vi "Begin.vi"() -> (0 "CameraDevRef 2":T1, 1 "CameraDevRef":T1)   [LabVIEW 2011]
doc: "Called before other user functions, this VI is expected to open initial I/O refnums, load in file data, and do all program initialization. Notice that the <B>error out</B> terminal is simply used for data flow. Wiring it to other structures or subVIs ensures that this VI runs first."
uses:
  <vilib>/Rock Robotics/WPI/Camera/WPI_CameraDevRef.ctl
  <vilib>/Rock Robotics/SystemInterfaces/DIO/FPGA_DIOPWMChannel.ctl
  <vilib>/Rock Robotics/WPI/Joystick/WPI_JoystickDeviceEnum.ctl
  <vilib>/Rock Robotics/SystemInterfaces/AI/FPGA_AIChannel.ctl
  <vilib>/Rock Robotics/SystemInterfaces/DIO/FPGA_DIORelayChannel.ctl
  <vilib>/Rock Robotics/SystemInterfaces/DIO/FPGA_DIOChannel.ctl
  <vilib>/Rock Robotics/SystemInterfaces/AI/FPGA_AIGyroChannel.ctl
  <vilib>/Rock Robotics/WPI/Relay/WPI_RelayDirection.ctl
  <vilib>/Rock Robotics/WPI/Encoder/WPI_EncoderType.ctl
  <vilib>/Rock Robotics/WPI/DriverStation/DriverStationLCD/WPI_DriverStationLCDLCDLine.ctl
  <vilib>/Rock Robotics/WPI/MotorControl/WPI_MotorControlOpen Victor.vi
  <vilib>/Rock Robotics/WPI/MotorControl/WPI_MotorControlOpen Jaguar.vi
  Robot Global Data.vi
  <vilib>/Utility/file.llb/Read From Spreadsheet File (DBL).vi
  <vilib>/Rock Robotics/WPI/Counter/WPI_CounterDigitalInputToDigitalSource.vi
  <vilib>/Rock Robotics/SystemInterfaces/Typedef/FPGA_TypedefDigitalModule.ctl
  <vilib>/Rock Robotics/SystemInterfaces/Typedef/FPGA_TypedefAnalogModule.ctl
panel:
  out "Path and file":string
  in  "Balls In Robot At Start":dbl=2.0
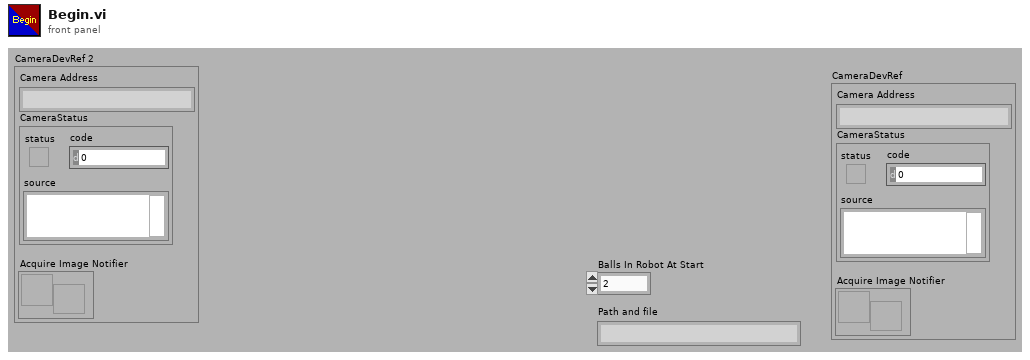
[diagram p1: front panel]
types:
  T1 = typedef "WPI_CameraDevRef.ctl" = cluster{"Camera Address":string, "CameraStatus":errorcluster, "Acquire Image Notifier":refnum<notifier>}
  T2 = typedef "FPGA_DIOPWMChannel.ctl" = enum8{"PWM 1", "PWM 2", "PWM 3", "PWM 4", "PWM 5", "PWM 6", "PWM 7", "PWM 8", "PWM 9", "PWM 10", "Invalid"}
  T3 = typedef "WPI_DriverStationLCDLCDLine.ctl" = enum16{"Main - Line 1", "User - Line 2", "User - Line 3", "User - Line 4", "User - Line 5", "User - Line 6"}
  T4 = typedef "WPI_EncoderType.ctl" = enum16{"1x", "2x", "4x"}
  T5 = typedef "FPGA_DIOChannel.ctl" = enum8{"DIO 1", "DIO 2", "DIO 3", "DIO 4", "DIO 5", "DIO 6", "DIO 7", "DIO 8", "DIO 9", "DIO 10", "DIO 11", "DIO 12", "DIO 13", "DIO 14", "Invalid"}
  T6 = typedef "FPGA_DIORelayChannel.ctl" = enum8{"Relay 1", "Relay 2", "Relay 3", "Relay 4", "Relay 5", "Relay 6", "Relay 7", "Relay 8", "Invalid"}
  T7 = typedef "WPI_RelayDirection.ctl" = enum16{"Both directions", "Forward only", "Reverse only"}
  T8 = typedef "FPGA_AIGyroChannel.ctl" = enum8{"AI 1", "AI 2", "Invalid"}
  T9 = typedef "FPGA_AIChannel.ctl" = enum8{"AI 1", "AI 2", "AI 3", "AI 4", "AI 5", "AI 6", "AI 7", "AI 8", "Invalid"}
  T10 = typedef "WPI_JoystickDeviceEnum.ctl" = enum16{"USB 1", "USB 2", "USB 3", "USB 4", "Kinect 1", "Kinect 2"}
  T11 = typedef "WPI_CameraImageSize.ctl" = enum16{"640x480", "320x240", "160x120"}
  T12 = cluster{"fps":i32, "compression":i32, "Image Size":T11}
  T13 = typedef "WPI_MotorControlDeviceRef.ctl" = cluster{"DeviceStatus":errorcluster, "Type":enum16{"PWM", "CAN"}, "PWM":cluster{"Digital Module":T14, "PWM Channel":T2, "DeadBand":T15}, "CAN":cluster{"Device Number":u8, "Control Mode":T16, "Semaphore":T17, "Max Vout":dbl}, "Invert":bool, "TransformRef":T18, "InvTransformRef":T18}
  T14 = typedef "FPGA_TypedefDigitalModule.ctl" = enum16{"Digital Module 1", "Digital Module 2"}
  T15 = typedef "WPI_PWMDeadband.ctl" = cluster{"Name":string, "maxPositivePwm":i32, "minPositivePwm":i32, "centerPwm":i32, "maxNegativePwm":i32, "minNegativePwm":i32, "angularRange":u16}
  T16 = typedef "WPI_CANJaguar_ControlMode.ctl" = enum8{"Percent VBus", "Current", "Speed", "Position", "Voltage"}
  T17 = typedef "Semaphore RefNum" = refnum<k1>
  T18 = typedef "WPI_PWMTransform_ConPane.ctl" = refnum<vi>
  T19 = typedef "WPI_ServoDeviceRef.ctl" = cluster{"DeviceStatus":errorcluster, "Digital Module":T14, "PWM Channel":T2, "DeadBand":T15}
  T20 = typedef "WPI_AnalogChannelDevRef.ctl" = cluster{"DevStatus":errorcluster, "Analog Module":T21, "Analog Channel":T9}
  T21 = typedef "FPGA_TypedefAnalogModule.ctl" = enum16{"Analog Module 1", "Analog Module 2"}
  T22 = typedef "WPI_CameraWhite Balance Values.ctl" = enum16{"Auto", "Fixed indoor", "Fixed outdoor 1", "Fixed outdoor 2", "Fixed fluorescent 1", "Fixed fluorescent 2", "Hold current"}
  T23 = typedef "WPI_JoystickDevRef.ctl" = cluster{"Device":T10}
  T24 = typedef "WPI_RelayDevRef.ctl" = cluster{"DevStatus":errorcluster, "Relay Channel":T6, "Digital Module":T14, "Relay Direction":T7}
  T25 = typedef "WPI_CameraExposure Values.ctl" = enum16{"Auto", "Flicker-free 50 Hz", "Flicker-free 60 Hz", "Hold current"}
  T26 = typedef "WPI_DigitalInputDevRef.ctl" = cluster{"DevStatus":errorcluster, "DIO Channel":T5, "Digital Module":T14}
  T27 = typedef "FPGA_CounterEncoderSourceConvertionLVSourceType.ctl" = cluster{"DevStatus":errorcluster, "AnalogTriggerMode?":bool, "DigitalMode":cluster{"Digital Module":T14, "DIO Channel":T28}, "AnalogTriggerMode":cluster{"AnalogTriggerIndex":T29, "OutputType":T30}}
  T28 = typedef "FPGA_DIODigitalSourceChannel.ctl" = enum8{"DIO 1", "DIO 2", "DIO 3", "DIO 4", "DIO 5", "DIO 6", "DIO 7", "DIO 8", "DIO 9", "DIO 10", "DIO 11", "DIO 12", "DIO 13", "DIO 14", "Disabled"}
  T29 = typedef "FPGA_AnalogTriggerIndex.ctl" = enum8{"Trig 0", "Trig 1", "Trig 2", "Trig 3", "Trig 4", "Trig 5", "Trig 6", "Trig 7", "Invalid"}
  T30 = typedef "FPGA_AnalogTriggerOutType.ctl" = enum16{"InWindow", "TriggerState", "Rising", "Falling"}
  T31 = typedef "WPI_EncoderDevRef.ctl" = cluster{"DevStatus":errorcluster, "EncoderIndex":T32, "CounterIndex":T33, "DistancePerCount":dbl, "Decoding Type":T4}
  T32 = typedef "FPGA_EncoderIdx.ctl" = enum8{"Enc 0", "Enc 1", "Enc 2", "Enc 3", "Invalid"}
  T33 = typedef "FPGA_CounterCtrSystemIndex.ctl" = enum8{"Ctr 0", "Ctr 1", "Ctr 2", "Ctr 3", "Ctr 4", "Ctr 5", "Ctr 6", "Ctr 7", "Invalid"}
  T34 = typedef "WPI_GyroDevRef.ctl" = cluster{"DevStatus":errorcluster, "Analog Module":T21, "Analog Channel":T9, "Offset":dbl, "Gain (VoltsPerDegree/Second)":dbl}
  T35 = typedef "WPI_UltrasonicDeviceRef.ctl" = cluster{"DevStatus":errorcluster, "Ping Digital Module":T14, "Echo Digital Module":T14, "Ping Channel":T5, "Echo Channel":T5, "CntIndex":T33}
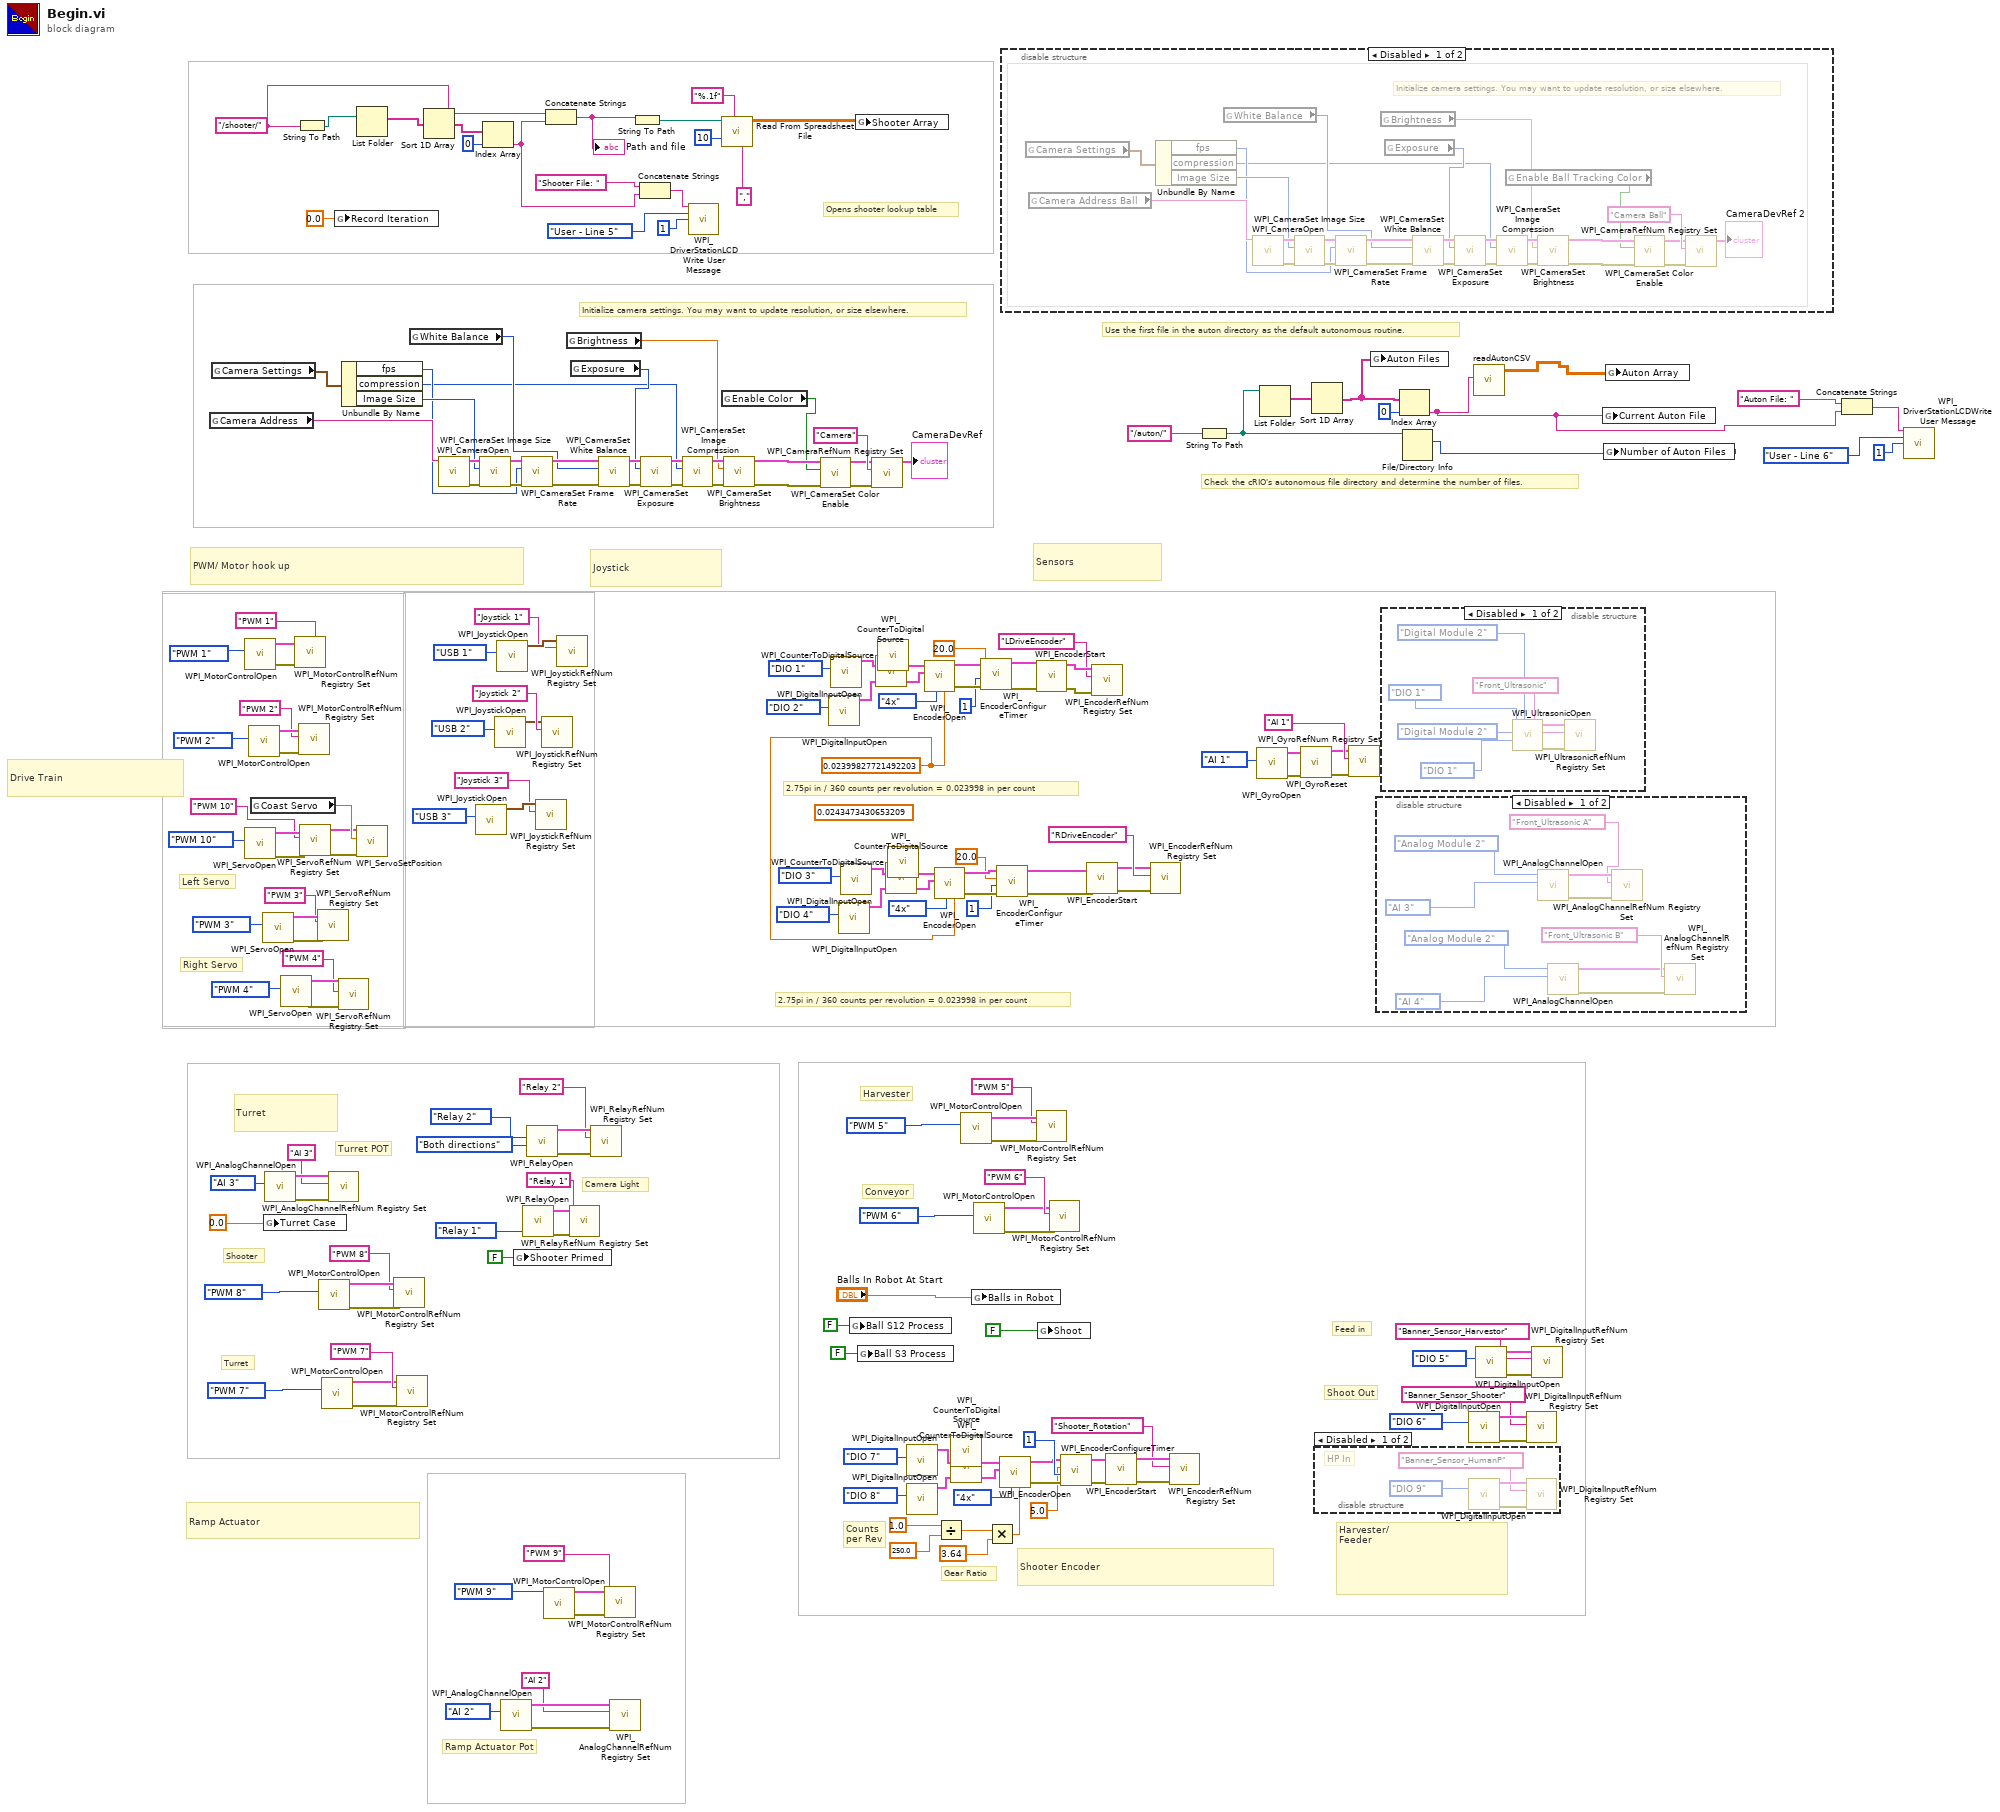
[diagram p0: block diagram]
diagram:
  (unwired) 0.0243473430653209 ("DistancePerCount")
  w39 = 0.02399827721492203 ("DistancePerCount")
  w87 = "/shooter/" ("string")
  # "Shooter Encoder"
  # "Counts\nper Rev"
  # "Gear Ratio"
  # "Check the cRIO's autonomous file directory and determine the number of files."
  # "Use the first file in the auton directory as the default autonomous routine."
  # "2.75pi in / 360 counts per revolution = 0.023998 in per count"
  # "2.75pi in / 360 counts per revolution = 0.023998 in per count"
  # "Opens shooter lookup table"
  # "Shoot Out"
  # "Feed in"
  # "Harvester"
  # "Conveyor"
  # "Shooter"
  # "Initialize camera settings. You may want to update resolution, or size elsewhere."
  # "Camera Light"
  # "Ramp Actuator Pot"
  # "Turret POT"
  # "Turret"
  # "Right Servo"
  # "Left Servo"
  # "Harvester/\nFeeder"
  # "Turret"
  # "Ramp Actuator"
  # "Drive Train"
  # "Sensors"
  # "Joystick"
  # "PWM/ Motor hook up"
  n1 = global read "Robot Global Data.vi" "Camera Address"() -> (w140:string)
  n2 = global read "Robot Global Data.vi" "Camera Settings"() -> (w139:T12)
  n3 = call-poly <vilib>:"WPI_MotorControlOpen.vi"("PWM Channel"=FPGA_DIOPWMChannel."PWM 1") -> ("error out"=w180:errorcluster, "MotorControlDeviceRef"=w182:T13)  [unwired: 9 in]
  n4 = call <vilib>:"WPI_ServoOpen.vi"("PWM Channel"=FPGA_DIOPWMChannel."PWM 10") -> ("error out"=w2:errorcluster, "ServoDeviceRef"=w6:T19)  [unwired: 9 in]
  n5 = call-poly <vilib>:"WPI_MotorControlOpen.vi"("PWM Channel"=FPGA_DIOPWMChannel."PWM 2") -> ("error out"=w178:errorcluster, "MotorControlDeviceRef"=w176:T13)  [unwired: 9 in]
  n6 = global read "Robot Global Data.vi" "Coast Servo"() -> (w7:dbl)
  n7 = call <vilib>:"WPI_ServoOpen.vi"("PWM Channel"=FPGA_DIOPWMChannel."PWM 3") -> ("error out"=w193:errorcluster, "ServoDeviceRef"=w198:T19)  [unwired: 9 in]
  n8 = global write "Robot Global Data.vi" "Turret Case"(0.0 ("Return To Home Case")) -> ()
  n9 = call <vilib>:"WPI_AnalogChannelOpen.vi"("Analog Channel"=FPGA_AIChannel."AI 3") -> ("error out"=w169:errorcluster, "AIDeviceRef"=w170:T20)  [unwired: 9 in]
  n10 = call <vilib>:"WPI_ServoOpen.vi"("PWM Channel"=FPGA_DIOPWMChannel."PWM 4") -> ("error out"=w192:errorcluster, "ServoDeviceRef"=w196:T19)  [unwired: 9 in]
  n11 = call <vilib>:"WPI_MotorControlRefNum Registry Set.vi"("error in (no error)"=w180, "refnum name"="PWM 1", "MotorControlDevRef"=w182) -> ()  [unwired: 7 in, 2 out]
  n12 = String To Path(string=w87) -> (path=w96:path)
  n13 = call <vilib>:"WPI_MotorControlRefNum Registry Set.vi"("error in (no error)"=w178, "refnum name"="PWM 2", "MotorControlDevRef"=w176) -> ()  [unwired: 7 in, 2 out]
  n14 = call <vilib>:"WPI_ServoRefNum Registry Set.vi"("error in (no error)"=w2, "refnum name"="PWM 10", "ServoDeviceRef"=w6) -> ("error out"=w3:errorcluster, "ServoDeviceRef"=w4:T19)  [unwired: 7 in]
  n15 = call <vilib>:"WPI_ServoRefNum Registry Set.vi"("error in (no error)"=w193, "refnum name"="PWM 3", "ServoDeviceRef"=w198) -> ()  [unwired: 7 in, 2 out]
  n16 = call-poly <vilib>:"WPI_MotorControlOpen.vi"("PWM Channel"=FPGA_DIOPWMChannel."PWM 8") -> ("error out"=w123:errorcluster, "MotorControlDeviceRef"=w125:T13)  [unwired: 9 in]
  n17 = call-poly <vilib>:"WPI_MotorControlOpen.vi"("PWM Channel"=FPGA_DIOPWMChannel."PWM 7") -> ("error out"=w174:errorcluster, "MotorControlDeviceRef"=w172:T13)  [unwired: 9 in]
  n18 = call <vilib>:"WPI_AnalogChannelRefNum Registry Set.vi"("error in (no error)"=w169, "refnum name"="AI 3", "AIDeviceRef"=w170) -> ()  [unwired: 7 in, 2 out]
  n19 = global write "Robot Global Data.vi" "Record Iteration"(0.0 ("Record Iteration")) -> ()
  n20 = call <vilib>:"WPI_ServoRefNum Registry Set.vi"("error in (no error)"=w192, "refnum name"="PWM 4", "ServoDeviceRef"=w196) -> ()  [unwired: 7 in, 2 out]
  n21 = Unbundle By Name(w139) -> ("fps"=w137:i32, "compression"=w134:i32, "Image Size"=w138:T11)
  n22 = List Folder(path=w96) -> (filenames=w95:string[])  [unwired: 1 in, 5 out]
  n23 = call <vilib>:"WPI_ServoSetPosition.vi"("error in (no error)"=w3, "Position"=w7, "ServoDeviceRef"=w4) -> ()  [unwired: 7 in, 2 out]
  n24 = call <vilib>:"WPI_MotorControlRefNum Registry Set.vi"("error in (no error)"=w123, "refnum name"="PWM 8", "MotorControlDevRef"=w125) -> ()  [unwired: 7 in, 2 out]
  n25 = call <vilib>:"WPI_MotorControlRefNum Registry Set.vi"("error in (no error)"=w174, "refnum name"="PWM 7", "MotorControlDevRef"=w172) -> ()  [unwired: 7 in, 2 out]
  n26 = global read "Robot Global Data.vi" "White Balance"() -> (w136:T22)
  n27 = Sort 1D Array(array=w95) -> (sorted array=w94:string[])
  n28 = call <vilib>:"WPI_CameraOpen.vi"("Camera Address"=w140) -> ("error out"=w146:errorcluster, "CameraDevRef"=w147:T1)  [unwired: 1 in, 8 out]
  n29 = call <vilib>:"WPI_JoystickOpen.vi"("JoystickDevice"=WPI_JoystickDeviceEnum."USB 3") -> ("JoystickDevRef"=w185:T23)  [unwired: 10 in]
  n30 = call <vilib>:"WPI_CameraSet Image Size.vi"("error in (no error)"=w146, "Image Size"=w138, "CameraDevRef"=w147) -> ("error out"=w145:errorcluster, "CameraDevRef Out"=w148:T1)  [unwired: 7 out]
  n31 = Index Array(array=w94, index=0) -> (element=w13:string)
  n32 = call <vilib>:"WPI_JoystickOpen.vi"("JoystickDevice"=WPI_JoystickDeviceEnum."USB 2") -> ("JoystickDevRef"=w188:T23)  [unwired: 10 in]
  n33 = call <vilib>:"WPI_JoystickOpen.vi"("JoystickDevice"=WPI_JoystickDeviceEnum."USB 1") -> ("JoystickDevRef"=w191:T23)  [unwired: 10 in]
  n34 = call <vilib>:"WPI_AnalogChannelOpen.vi"("Analog Channel"=FPGA_AIChannel."AI 2") -> ("error out"=w164:errorcluster, "AIDeviceRef"=w165:T20)  [unwired: 9 in]
  n35 = global write "Robot Global Data.vi" "Shooter Primed"(FALSE ("Ball S3 Process")) -> ()
  n36 = call <vilib>:"WPI_CameraSet Frame Rate.vi"("error in (no error)"=w145, "Frame Rate (fps)"=w137, "CameraDevRef"=w148) -> ("error out"=w144:errorcluster, "CameraDevRef Out"=w150:T1)  [unwired: 7 out]
  n37 = call <vilib>:"WPI_RelayOpen.vi"("Relay Channel"=FPGA_DIORelayChannel."Relay 1") -> ("error out"=w157:errorcluster, "RelayDevRef"=w156:T24)  [unwired: 9 in]
  n38 = call <vilib>:"WPI_RelayOpen.vi"("Relay Direction"=WPI_RelayDirection."Both directions", "Relay Channel"=FPGA_DIORelayChannel."Relay 2") -> ("error out"=w82:errorcluster, "RelayDevRef"=w83:T24)  [unwired: 8 in]
  n39 = call <vilib>:"WPI_JoystickRefNum Registry Set.vi"("refnum name"="Joystick 3", "JoystickDevRef"=w185) -> ()  [unwired: 8 in, 2 out]
  n40 = call <vilib>:"WPI_JoystickRefNum Registry Set.vi"("refnum name"="Joystick 2", "JoystickDevRef"=w188) -> ()  [unwired: 8 in, 2 out]
  n41 = call-poly <vilib>:"WPI_MotorControlOpen.vi"("PWM Channel"=FPGA_DIOPWMChannel."PWM 9") -> ("error out"=w160:errorcluster, "MotorControlDeviceRef"=w161:T13)  [unwired: 9 in]
  n42 = Concatenate Strings(w87, w13) -> (w89:string)
  "Path and file" <- w89
  n43 = call <vilib>:"WPI_JoystickRefNum Registry Set.vi"("refnum name"="Joystick 1", "JoystickDevRef"=w191) -> ()  [unwired: 8 in, 2 out]
  n44 = global read "Robot Global Data.vi" "Brightness"() -> (w133:dbl)
  n45 = call <vilib>:"WPI_RelayRefNum Registry Set.vi"("error in (no error)"=w157, "refnum name"="Relay 1", "RelayDevRef"=w156) -> ()  [unwired: 7 in, 2 out]
  n46 = global read "Robot Global Data.vi" "Exposure"() -> (w135:T25)
  n47 = call <vilib>:"WPI_RelayRefNum Registry Set.vi"("error in (no error)"=w82, "refnum name"="Relay 2", "RelayDevRef"=w83) -> ()  [unwired: 7 in, 2 out]
  n48 = call <vilib>:"WPI_CameraSet White Balance.vi"("error in (no error)"=w144, "White Balance"=w136, "CameraDevRef"=w150) -> ("error out"=w143:errorcluster, "CameraDevRef Out"=w149:T1)  [unwired: 7 out]
  n49 = call <vilib>:"WPI_MotorControlRefNum Registry Set.vi"("error in (no error)"=w160, "refnum name"="PWM 9", "MotorControlDevRef"=w161) -> ()  [unwired: 7 in, 2 out]
  n50 = call <vilib>:"WPI_AnalogChannelRefNum Registry Set.vi"("error in (no error)"=w164, "refnum name"="AI 2", "AIDeviceRef"=w165) -> ()  [unwired: 7 in, 2 out]
  n51 = String To Path(string=w89) -> (path=w88:path)
  n52 = Concatenate Strings("Shooter File: ", w13) -> (w11:string)
  n53 = call <vilib>:"WPI_CameraSet Exposure.vi"("error in (no error)"=w143, "Exposure"=w135, "CameraDevRef"=w149) -> ("error out"=w142:errorcluster, "CameraDevRef Out"=w152:T1)  [unwired: 7 out]
  n54 = call <vilib>:"WPI_CameraSet Image Compression.vi"("error in (no error)"=w142, "Compression"=w134, "CameraDevRef"=w152) -> ("error out"=w141:errorcluster, "CameraDevRef Out"=w151:T1)  [unwired: 7 out]
  n55 = call <vilib>:"WPI_DriverStationLCDWrite User Message.vi"("line text"=w11, "line"=WPI_DriverStationLCDLCDLine."User - Line 5", "starting column"=i8 1) -> ()  [unwired: 2 in, 11 out]
  n56 = call-poly <vilib>:"Read From Spreadsheet File.vi"("delimiter (\\t)"="," ("delimiter (\\t)"), "format (%.3f)"="%.1f", "number of rows (all:-1)"=10, "file path (dialog if empty)"=w88) -> ("all rows"=w86:dbl[][])  [unwired: 1 in, 6 out]
  n57 = global read "Robot Global Data.vi" "Enable Color"() -> (w128:bool)
  n58 = call <vilib>:"WPI_CameraSet Brightness.vi"("error in (no error)"=w141, "Brightness"=w133, "CameraDevRef"=w151) -> ("error out"=w131:errorcluster, "CameraDevRef Out"=w132:T1)  [unwired: 7 out]
  n59 = call <vilib>:"WPI_CameraSet Color Enable.vi"("error in (no error)"=w131, "Color Enabled"=w128, "CameraDevRef"=w132) -> ("error out"=w129:errorcluster, "CameraDevRef Out"=w130:T1)  [unwired: 7 in]
  n60 = call <vilib>:"WPI_DigitalInputOpen.vi"("DIO Channel"=FPGA_DIOChannel."DIO 2") -> ("DigitalInputDevRef"=w74:T26)  [unwired: 9 in, 1 out]
  n61 = call <vilib>:"WPI_DigitalInputOpen.vi"("DIO Channel"=FPGA_DIOChannel."DIO 1") -> ("DigitalInputDevRef"=w71:T26)  [unwired: 9 in, 1 out]
  n62 = call <vilib>:"WPI_DigitalInputOpen.vi"("DIO Channel"=FPGA_DIOChannel."DIO 4") -> ("DigitalInputDevRef"=w65:T26)  [unwired: 9 in, 1 out]
  n63 = call <vilib>:"WPI_DigitalInputOpen.vi"("DIO Channel"=FPGA_DIOChannel."DIO 3") -> ("DigitalInputDevRef"=w68:T26)  [unwired: 9 in, 1 out]
  n64 = global write "Robot Global Data.vi" "Ball S12 Process"(FALSE ("Ball S12 Process")) -> ()
  n65 = global write "Robot Global Data.vi" "Shooter Array"(w86) -> ()
  n66 = global write "Robot Global Data.vi" "Ball S3 Process"(FALSE ("Ball S3 Process")) -> ()
  n67 = call <vilib>:"WPI_CameraRefNum Registry Set.vi"("error in (no error)"=w129, "refnum name"="Camera", "CameraDevRef"=w130) -> ("CameraDevRef"=→"CameraDevRef":T1)  [unwired: 8 out]
  n68 = call-poly <vilib>:"WPI_CounterToDigitalSource.vi"("DigitalInputDevRef"=w74) -> ("Digital Source"=w75:T27)  [unwired: 6 in]
  n69 = call-poly <vilib>:"WPI_CounterToDigitalSource.vi"("DigitalInputDevRef"=w71) -> ("Digital Source"=w70:T27)  [unwired: 6 in]
  n70 = call-poly <vilib>:"WPI_CounterToDigitalSource.vi"("DigitalInputDevRef"=w65) -> ("Digital Source"=w64:T27)  [unwired: 6 in]
  n71 = call-poly <vilib>:"WPI_CounterToDigitalSource.vi"("DigitalInputDevRef"=w68) -> ("Digital Source"=w69:T27)  [unwired: 6 in]
  n72 = call <vilib>:"WPI_DigitalInputOpen.vi"("DIO Channel"=FPGA_DIOChannel."DIO 7") -> ("DigitalInputDevRef"=w23:T26)  [unwired: 9 in, 1 out]
  n73 = call <vilib>:"WPI_DigitalInputOpen.vi"("DIO Channel"=FPGA_DIOChannel."DIO 8") -> ("DigitalInputDevRef"=w26:T26)  [unwired: 9 in, 1 out]
  n74 = call <vilib>:"WPI_EncoderOpen.vi"("DistancePerCount"=w39, "Decoding Type"=WPI_EncoderType."4x", "BSource"=w75, "ASource"=w70) -> ("error out"=w43:errorcluster, "EncoderDevRef"=w46:T31)  [unwired: 6 in]
  n75 = call <vilib>:"WPI_EncoderOpen.vi"("DistancePerCount"=w39, "Decoding Type"=WPI_EncoderType."4x", "BSource"=w64, "ASource"=w69) -> ("error out"=w61:errorcluster, "EncoderDevRef"=w60:T31)  [unwired: 6 in]
  n76 = Divide(x=1.0, y=250.0) -> (x/y=w20:dbl)
  n77 = call-poly <vilib>:"WPI_CounterToDigitalSource.vi"("DigitalInputDevRef"=w23) -> ("Digital Source"=w22:T27)  [unwired: 6 in]
  n78 = call-poly <vilib>:"WPI_CounterToDigitalSource.vi"("DigitalInputDevRef"=w26) -> ("Digital Source"=w27:T27)  [unwired: 6 in]
  n79 = call-poly <vilib>:"WPI_MotorControlOpen.vi"("PWM Channel"=FPGA_DIOPWMChannel."PWM 5") -> ("error out"=w119:errorcluster, "MotorControlDeviceRef"=w121:T13)  [unwired: 9 in]
  n80 = global write "Robot Global Data.vi" "Balls in Robot"("Balls In Robot At Start") -> ()
  n81 = call-poly <vilib>:"WPI_MotorControlOpen.vi"("PWM Channel"=FPGA_DIOPWMChannel."PWM 6") -> ("error out"=w118:errorcluster, "MotorControlDeviceRef"=w116:T13)  [unwired: 9 in]
  n82 = call <vilib>:"WPI_EncoderConfigureTimer.vi"("error in (no error)"=w43, "Number Samples to Average"=u8 1, "Minimum Rate"=20.0, "EncoderDevRef"=w46) -> ("error out"=w44:errorcluster, "EncoderDevRef"=w45:T31)  [unwired: 6 in]
  n83 = Multiply(x=w20, y=3.64) -> (x*y=w18:dbl)
  n84 = call <vilib>:"WPI_EncoderConfigureTimer.vi"("error in (no error)"=w61, "Number Samples to Average"=u8 1, "Minimum Rate"=20.0, "EncoderDevRef"=w60) -> ("error out"=w57:errorcluster, "EncoderDevRef"=w58:T31)  [unwired: 6 in]
  n85 = call <vilib>:"WPI_EncoderOpen.vi"("DistancePerCount"=w18, "Decoding Type"=WPI_EncoderType."4x", "BSource"=w27, "ASource"=w22) -> ("error out"=w30:errorcluster, "EncoderDevRef"=w31:T31)  [unwired: 6 in]
  n86 = disable-structure shown="Disabled" {
    frame Disabled {
      # "Initialize camera settings. You may want to update resolution, or size elsewhere."
      n87 = global read "Robot Global Data.vi" "Camera Settings"() -> (w212:T12)
      n88 = global read "Robot Global Data.vi" "Camera Address Ball"() -> (w213:string)
      n89 = Unbundle By Name(w212) -> ("fps"=w210:i32, "compression"=w207:i32, "Image Size"=w211:T11)
      n90 = global read "Robot Global Data.vi" "White Balance"() -> (w209:T22)
      n91 = call <vilib>:"WPI_CameraOpen.vi"("Camera Address"=w213) -> ("error out"=w219:errorcluster, "CameraDevRef"=w220:T1)  [unwired: 1 in, 8 out]
      n92 = call <vilib>:"WPI_CameraSet Image Size.vi"("error in (no error)"=w219, "Image Size"=w211, "CameraDevRef"=w220) -> ("error out"=w218:errorcluster, "CameraDevRef Out"=w221:T1)  [unwired: 7 out]
      n93 = call <vilib>:"WPI_CameraSet Frame Rate.vi"("error in (no error)"=w218, "Frame Rate (fps)"=w210, "CameraDevRef"=w221) -> ("error out"=w217:errorcluster, "CameraDevRef Out"=w223:T1)  [unwired: 7 out]
      n94 = global read "Robot Global Data.vi" "Brightness"() -> (w206:dbl)
      n95 = global read "Robot Global Data.vi" "Exposure"() -> (w208:T25)
      n96 = call <vilib>:"WPI_CameraSet White Balance.vi"("error in (no error)"=w217, "White Balance"=w209, "CameraDevRef"=w223) -> ("error out"=w216:errorcluster, "CameraDevRef Out"=w222:T1)  [unwired: 7 out]
      n97 = call <vilib>:"WPI_CameraSet Exposure.vi"("error in (no error)"=w216, "Exposure"=w208, "CameraDevRef"=w222) -> ("error out"=w215:errorcluster, "CameraDevRef Out"=w225:T1)  [unwired: 7 out]
      n98 = call <vilib>:"WPI_CameraSet Image Compression.vi"("error in (no error)"=w215, "Compression"=w207, "CameraDevRef"=w225) -> ("error out"=w214:errorcluster, "CameraDevRef Out"=w224:T1)  [unwired: 7 out]
      n99 = global read "Robot Global Data.vi" "Enable Ball Tracking Color"() -> (w201:bool)
      n100 = call <vilib>:"WPI_CameraSet Brightness.vi"("error in (no error)"=w214, "Brightness"=w206, "CameraDevRef"=w224) -> ("error out"=w204:errorcluster, "CameraDevRef Out"=w205:T1)  [unwired: 7 out]
      n101 = call <vilib>:"WPI_CameraSet Color Enable.vi"("error in (no error)"=w204, "Color Enabled"=w201, "CameraDevRef"=w205) -> ("error out"=w202:errorcluster, "CameraDevRef Out"=w203:T1)  [unwired: 7 in]
      n102 = call <vilib>:"WPI_CameraRefNum Registry Set.vi"("error in (no error)"=w202, "refnum name"="Camera Ball", "CameraDevRef"=w203) -> ("CameraDevRef"=→"CameraDevRef 2":T1)  [unwired: 8 out]
    }
    frame Enabled {
    }
  }
  n103 = call <vilib>:"WPI_EncoderStart.vi"("error in (no error)"=w44, "EncoderDevRef"=w45) -> ("error out"=w78:errorcluster, "EncoderDevRef"=w77:T31)  [unwired: 8 in]
  n104 = call <vilib>:"WPI_MotorControlRefNum Registry Set.vi"("error in (no error)"=w119, "refnum name"="PWM 5", "MotorControlDevRef"=w121) -> ()  [unwired: 7 in, 2 out]
  n105 = global write "Robot Global Data.vi" "Shoot"(FALSE ("Ball S12 Process")) -> ()
  n106 = call <vilib>:"WPI_MotorControlRefNum Registry Set.vi"("error in (no error)"=w118, "refnum name"="PWM 6", "MotorControlDevRef"=w116) -> ()  [unwired: 7 in, 2 out]
  n107 = call <vilib>:"WPI_EncoderConfigureTimer.vi"("error in (no error)"=w30, "Number Samples to Average"=u8 1, "Minimum Rate"=5.0, "EncoderDevRef"=w31) -> ("error out"=w34:errorcluster, "EncoderDevRef"=w33:T31)  [unwired: 6 in]
  n108 = call <vilib>:"WPI_EncoderStart.vi"("error in (no error)"=w57, "EncoderDevRef"=w58) -> ("error out"=w55:errorcluster, "EncoderDevRef"=w56:T31)  [unwired: 8 in]
  n109 = call <vilib>:"WPI_EncoderRefNum Registry Set.vi"("error in (no error)"=w78, "refnum name"="LDriveEncoder", "EncoderDevRef"=w77) -> ()  [unwired: 7 in, 2 out]
  n110 = call <vilib>:"WPI_EncoderStart.vi"("error in (no error)"=w34, "EncoderDevRef"=w33) -> ("error out"=w36:errorcluster, "EncoderDevRef"=w35:T31)  [unwired: 8 in]
  n111 = call <vilib>:"WPI_EncoderRefNum Registry Set.vi"("error in (no error)"=w55, "refnum name"="RDriveEncoder", "EncoderDevRef"=w56) -> ()  [unwired: 7 in, 2 out]
  n112 = call <vilib>:"WPI_EncoderRefNum Registry Set.vi"("error in (no error)"=w36, "refnum name"="Shooter_Rotation", "EncoderDevRef"=w35) -> ()  [unwired: 7 in, 2 out]
  n113 = String To Path(string="/auton/") -> (path=w51:path)
  n114 = call <vilib>:"WPI_GyroOpen.vi"("Analog Channel"=FPGA_AIGyroChannel."AI 1") -> ("error out"=w99:errorcluster, "GyroDevRef"=w100:T34)  [unwired: 8 in, 1 out]
  n115 = List Folder(path=w51) -> (filenames=w50:string[])  [unwired: 1 in, 5 out]
  n116 = call <vilib>:"WPI_GyroReset.vi"("error in (no error)"=w99, "GyroDevRef"=w100) -> ("error out"=w98:errorcluster, "GyroDevRef"=w97:T34)  [unwired: 8 in]
  n117 = Sort 1D Array(array=w50) -> (sorted array=w48:string[])
  n118 = disable-structure shown="Disabled" {
    frame Disabled {
      # "HP In"
      n119 = call <vilib>:"WPI_DigitalInputOpen.vi"("DIO Channel"=FPGA_DIOChannel."DIO 9") -> ("error out"=w229:errorcluster, "DigitalInputDevRef"=w228:T26)  [unwired: 9 in]
      n120 = call <vilib>:"WPI_DigitalInputRefNum Registry Set.vi"("error in (no error)"=w229, "refnum name"="Banner_Sensor_HumanP", "DigitalInputDevRef"=w228) -> ()  [unwired: 7 in, 2 out]
    }
    frame Enabled {
    }
  }
  n121 = call <vilib>:"WPI_GyroRefNum Registry Set.vi"("error in (no error)"=w98, "refnum name"="AI 1", "GyroDevRef"=w97) -> ()  [unwired: 7 in, 2 out]
  n122 = global write "Robot Global Data.vi" "Auton Files"(w48) -> ()
  n123 = disable-structure shown="Disabled" {
    frame Disabled {
      n124 = call <vilib>:"WPI_AnalogChannelOpen.vi"("Analog Channel"=FPGA_AIChannel."AI 3", "Analog Module (Module 1)"=FPGA_TypedefAnalogModule."Analog Module 2") -> ("error out"=w236:errorcluster, "AIDeviceRef"=w235:T20)  [unwired: 8 in]
      n125 = call <vilib>:"WPI_AnalogChannelOpen.vi"("Analog Channel"=FPGA_AIChannel."AI 4", "Analog Module (Module 1)"=FPGA_TypedefAnalogModule."Analog Module 2") -> ("error out"=w231:errorcluster, "AIDeviceRef"=w232:T20)  [unwired: 8 in]
      n126 = call <vilib>:"WPI_AnalogChannelRefNum Registry Set.vi"("error in (no error)"=w236, "refnum name"="Front_Ultrasonic A", "AIDeviceRef"=w235) -> ()  [unwired: 7 in, 2 out]
      n127 = call <vilib>:"WPI_AnalogChannelRefNum Registry Set.vi"("error in (no error)"=w231, "refnum name"="Front_Ultrasonic B", "AIDeviceRef"=w232) -> ()  [unwired: 7 in, 2 out]
    }
    frame Enabled {
    }
  }
  n128 = disable-structure shown="Disabled" {
    frame Disabled {
      n129 = call <vilib>:"WPI_UltrasonicOpen.vi"("Ping Digital Module (Module 1)"=FPGA_TypedefDigitalModule."Digital Module 2", "Echo DIO Channel"=FPGA_DIOChannel."DIO 1", "Echo Digital Module (Module 1)"=FPGA_TypedefDigitalModule."Digital Module 2", "Ping DIO Channel"=FPGA_DIOChannel."DIO 1") -> ("error out"=w247:errorcluster, "UltrasonicDevRef"=w246:T35)  [unwired: 6 in]
      n130 = call <vilib>:"WPI_UltrasonicRefNum Registry Set.vi"("error in (no error)"=w247, "refnum name"="Front_Ultrasonic", "UltrasonicDevRef"=w246) -> ()  [unwired: 7 in, 2 out]
    }
    frame Enabled {
    }
  }
  n131 = Index Array(array=w48, index=0) -> (element=w9:string)
  n132 = File/Directory Info(path=w51) -> (size=w53:i64)  [unwired: 1 in, 6 out]
  n133 = call <vilib>:"WPI_DigitalInputOpen.vi"("DIO Channel"=FPGA_DIOChannel."DIO 6") -> ("error out"=w109:errorcluster, "DigitalInputDevRef"=w108:T26)  [unwired: 9 in]
  n134 = call "readAutonCSV.vi"("AutonFile"=w9) -> ("AutonArray"=w47:dbl[][])  [unwired: 7 in]
  n135 = call <vilib>:"WPI_DigitalInputOpen.vi"("DIO Channel"=FPGA_DIOChannel."DIO 5") -> ("error out"=w112:errorcluster, "DigitalInputDevRef"=w111:T26)  [unwired: 9 in]
  n136 = call <vilib>:"WPI_DigitalInputRefNum Registry Set.vi"("error in (no error)"=w109, "refnum name"="Banner_Sensor_Shooter", "DigitalInputDevRef"=w108) -> ()  [unwired: 7 in, 2 out]
  n137 = call <vilib>:"WPI_DigitalInputRefNum Registry Set.vi"("error in (no error)"=w112, "refnum name"="Banner_Sensor_Harvestor", "DigitalInputDevRef"=w111) -> ()  [unwired: 7 in, 2 out]
  n138 = global write "Robot Global Data.vi" "Current Auton File"(w9) -> ()
  n139 = global write "Robot Global Data.vi" "Number of Auton Files"(w53) -> ()
  n140 = global write "Robot Global Data.vi" "Auton Array"(w47) -> ()
  n141 = Concatenate Strings("Auton File: ", w9) -> (w8:string)
  n142 = call <vilib>:"WPI_DriverStationLCDWrite User Message.vi"("line text"=w8, "line"=WPI_DriverStationLCDLCDLine."User - Line 6", "starting column"=i8 1) -> ()  [unwired: 2 in, 11 out]
